vi "After Iterative Read.vi"(8 "Error In":errorcluster, 10 "Local File":refnum<file>, 11 "SFTP File":refnum<class "SFTP File.lvclass">) -> (0 "Error Out":errorcluster, 2 "Remote Path":string, 3 "SFTP":refnum<class "SFTP.lvclass">)   [LabVIEW 2018, in "Tests.lvlib" / "SFTP File.lvlib"]
uses:
  SFTP File.lvlib
  src/Toolkit/SFTP File/SFTP File.lvclass
  src/Toolkit/SFTP/SFTP.lvclass
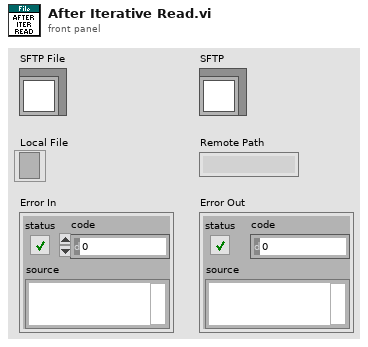
[diagram p1: front panel]
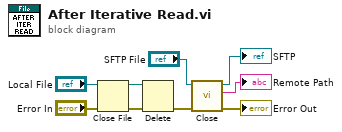
[diagram p0: block diagram]
diagram:
  n1 = Close File(refnum="Local File", error in="Error In") -> (path=w2:path, error out=w5:errorcluster)
  n2 = Delete(path (use dialog)=w2, error in=w5) -> (error out=w1:errorcluster)  [unwired: 3 in, 2 out]
  n3 = call "Close.vi"("Error In"=w1, "SFTP File"="SFTP File") -> ("Error Out"=→"Error Out":errorcluster, "Remote Path"=→"Remote Path":string, "SFTP"=→"SFTP":refnum<class "SFTP.lvclass">)  [unwired: 7 in]
